vi "Historical Error (SubVI).vi"(6 "in":bool, 10 "Warnings bool array":bool[](array[boolean]), 11 "error table in":T1(array[cluster]) {"Time Stamp" format="%<%.3X %x>T"}) -> (3 "error table out":T1(array[cluster]) {"Time Stamp" format="%<%.3X %x>T"})   [LabVIEW 2022 SP3]
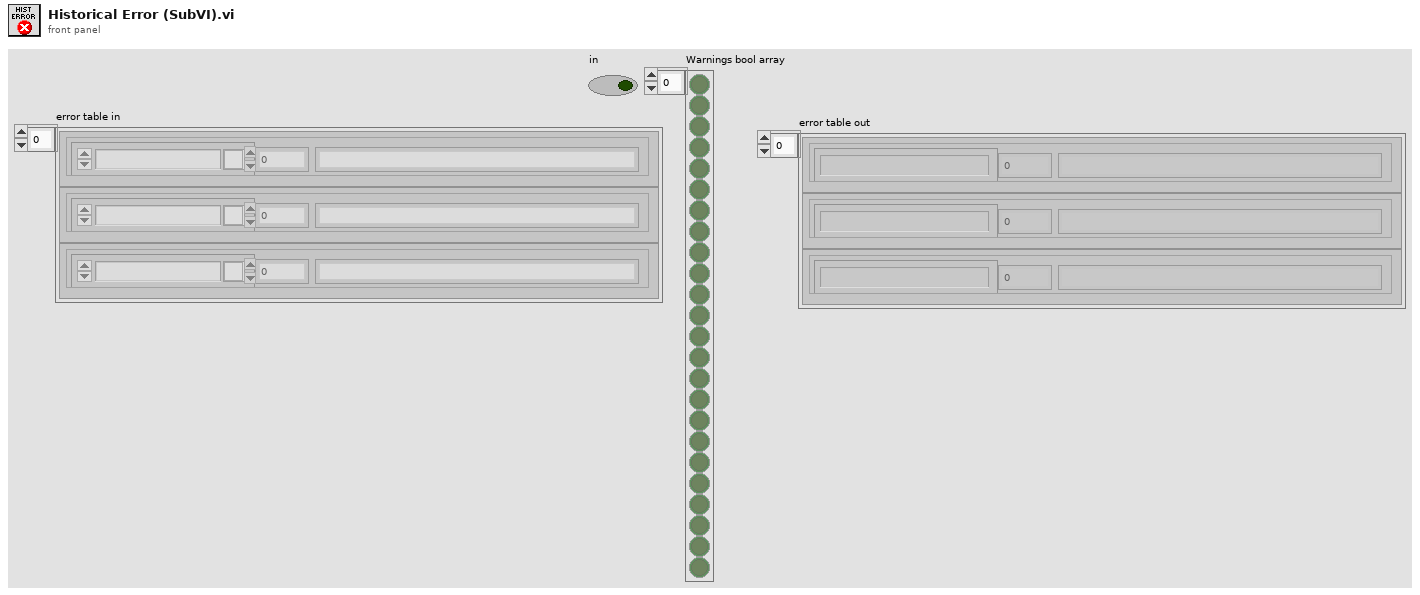
[diagram p1: front panel]
types:
  T1 = cluster{"Time Stamp":timestamp, "Descripcion":string, "Numeric":i32}[]
  T2 = cluster{"Time Stamp":timestamp, "Descripcion":string, "Numeric":i32}
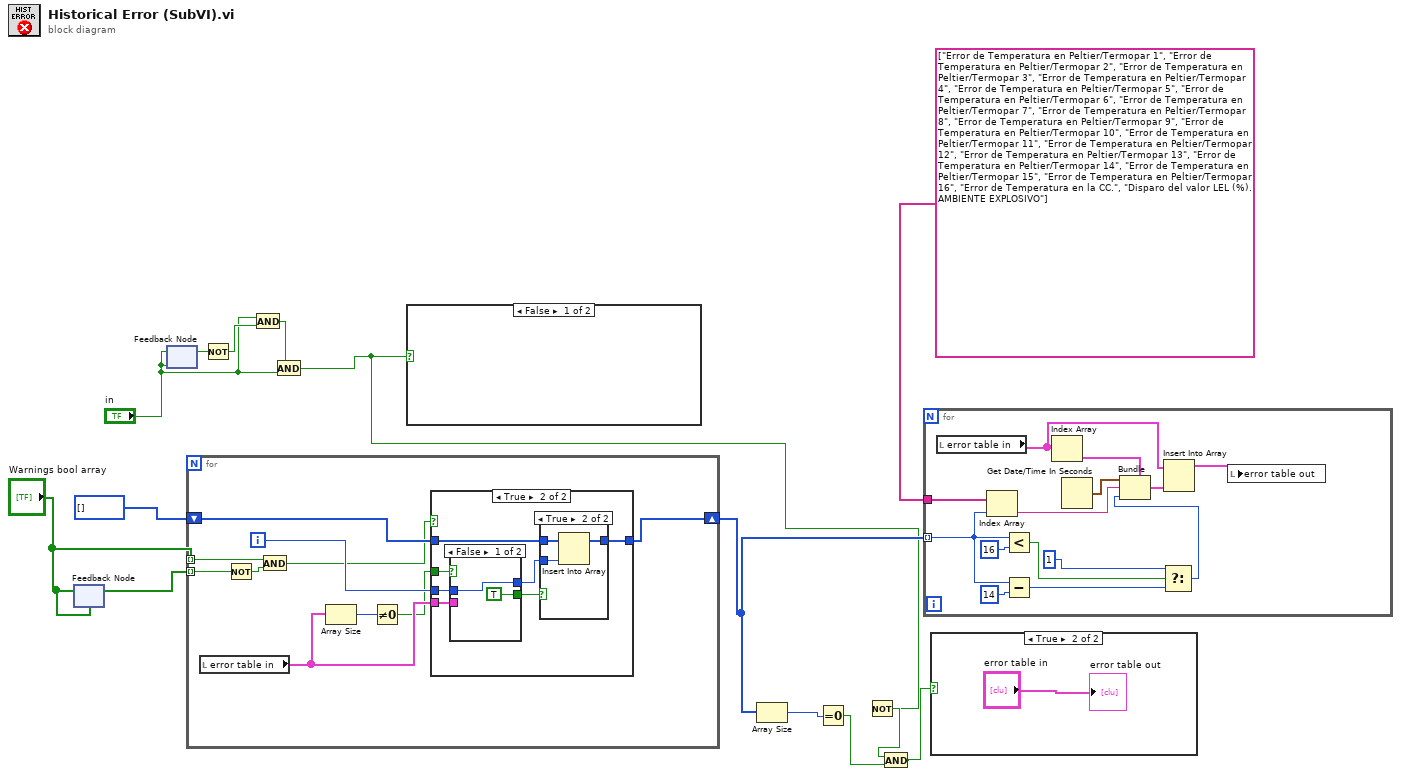
[diagram p0: block diagram]
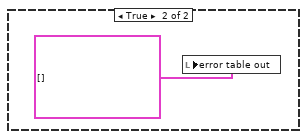
[diagram p3: hidden frame]
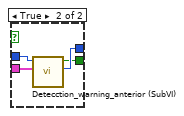
[diagram p5: hidden frame]
diagram:
  n1 = feedback #1("Warnings bool array") -> (w11:bool[])
  n2 = feedback-in #1("Warnings bool array") -> ()
  n3 = feedback #2("in") -> (w7:bool)
  n4 = feedback-in #2("in") -> ()
  n5 = for {
    tunnel: w11 -> [w24] mode=indexing
    tunnel: "Warnings bool array" -> [w22] mode=indexing
    shift-right: [w19] -> w10
    shift-left: i32[] [] -> [w21]
    i -> [w20]
    n6 = local read "error table in"() -> (w18:T1)
    n7 = Not(x=w24) -> (.not. x?=w23:bool)
    n8 = And(x=w22, y=w23) -> (x .and. y?=w16:bool)
    n9 = Array Size(array=w18) -> (size(s)=w17:i32)
    n10 = Not Equal To 0?(x=w17) -> (x != 0?=w15:bool)
    n11 = case shown="True" w16 {
      tunnel: w21 -> [w25 w32]
      tunnel: w20 -> [_ w30]
      tunnel: [w25 w31] -> w19
      tunnel: w18 -> [_ w27]
      tunnel: w15 -> [_ w26]
      frame False {
      }
      frame True {
        n12 = case shown="False" w26 {
          tunnel: w30 -> [w33 w38]
          tunnel: [w33 w37] -> w29
          tunnel: [TRUE ("Add W?") w36] -> w28
          tunnel: w27 -> [_ w35]
          frame False {
          }
          frame True {
            n13 = call "Detecction_warning_anterior (SubVI).vi"("warnings table in"=w35, "Index in"=w38) -> ("Index Out"=w37:i32, "Add W?"=w36:bool)  [unwired: 8 in]
          }
        }
        n14 = case shown="True" w28 {
          tunnel: w32 -> [w39 w42]
          tunnel: [w39 w41] -> w31
          tunnel: w29 -> [_ w40]
          frame False {
          }
          frame True {
            n15 = Insert Into Array(array=w42, new element=w40) -> (w41:i32[])  [unwired: 1 in]
          }
        }
      }
    }
  }
  n16 = Not(x=w7) -> (.not. x?=w8:bool)
  n17 = And(x="in", y=w8) -> (x .and. y?=w6:bool)
  n18 = And(x=w6, y="in") -> (x .and. y?=w2:bool)
  n19 = case shown="False" w2 {
    frame False {
    }
    frame True {
      n20 = local write "error table out"(T1 [] ("Warnings table out")) -> ()
    }
  }
  n21 = Array Size(array=w10) -> (size(s)=w9:i32)
  n22 = Equal To 0?(x=w9) -> (x = 0?=w4:bool)
  n23 = Not(x=w2) -> (.not. x?=w3:bool)
  n24 = And(x=w3, y=w4) -> (x .and. y?=w1:bool)
  n25 = for {
    tunnel: w10 -> [w46] mode=indexing
    tunnel: string[] ["Error de Temperatura en Peltier/Termopar 1", "Error de Temperatura en Peltier/Termopar 2", "Error de Temperatura en Peltier/Termopar 3", "Error de Temperatura en Peltier/Termopar 4", "Error de Temperatura en Peltier/Termopar 5", "Error de Temperatura en Peltier/Termopar 6", "Error de Temperatura en Peltier/Termopar 7", "Error de Temperatura en Peltier/Termopar 8", "Error de Temperatura en Peltier/Termopar 9", "Error de Temperatura en Peltier/Termopar 10", "Error de Temperatura en Peltier/Termopar 11", "Error de Temperatura en Peltier/Termopar 12", "Error de Temperatura en Peltier/Termopar 13", "Error de Temperatura en Peltier/Termopar 14", "Error de Temperatura en Peltier/Termopar 15", "Error de Temperatura en Peltier/Termopar 16", "Error de Temperatura en la CC.", "Disparo del valor LEL (%). AMBIENTE EXPLOSIVO"] -> [w54]
    n26 = local read "error table in"() -> (w44:T1)
    n27 = Index Array(array=w54, index=w46) -> (element=w53:string)
    n28 = Less?(x=w46, y=16) -> (x < y?=w51:bool)
    n29 = Subtract(x=w46, y=14) -> (x-y=w48:i32)
    n30 = Index Array(array=w44) -> (element=w56:T2)  [unwired: 1 in]
    n31 = Get Date/Time In Seconds() -> (seconds since 1Jan1904=w55:timestamp)
    n32 = Select(t=1, s=w51, f=w48) -> (s? t:f=w47:i32)
    n33 = Bundle(cluster=w56, "Time Stamp"=w55, "Descripcion"=w53, "Numeric"=w47) -> (w57:T2)
    n34 = Insert Into Array(array=w44, new element=w57) -> (w45:T1)  [unwired: 1 in]
    n35 = local write "error table out"(w45) -> ()
  }
  n36 = case shown="True" w1 {
    frame False {
    }
    frame True {
      "error table out" <- "error table in"
    }
  }
